vi "DSF.Transceiver.UDP.Get Transfer Group Parameters.vi"(11 "UDP Transceiver in":refnum<class "DSF.Transceiver.UDP.lvclass">) -> (2 "Transfer Group parameters":T1[](array[typedef]) {"Rx"."max size" format="%d bytes"; "Rx"."Transfers Rx"."timeout" format="%d ms"; "Rx"."Transfers Rx"."max size" format="%d bytes"}, 3 "UDP Transceiver out":refnum<class "DSF.Transceiver.UDP.lvclass">)   [LabVIEW 2017, in "DSF.Transceiver.UDP.lvlib" / "DSF.Transceiver.UDP.lvclass"]
uses:
  DSF.Transceiver.UDP.lvclass
  DSF.Transceiver.UDP.Parameters.Transfer Group.ctl
  DSF.Transceiver.UDP.Parameters.Transfer Group.Rx.ctl
  DSF.Transceiver.UDP.Parameters.Transfer.Rx.ctl
  DSF.Transceiver.UDP.Parameters.Transfer Group.Tx.ctl
  DSF.Transceiver.UDP.Parameters.Transfer.Tx.ctl
  DSF.Transceiver.UDP.lvclass/DSF.Transceiver.UDP.ctl
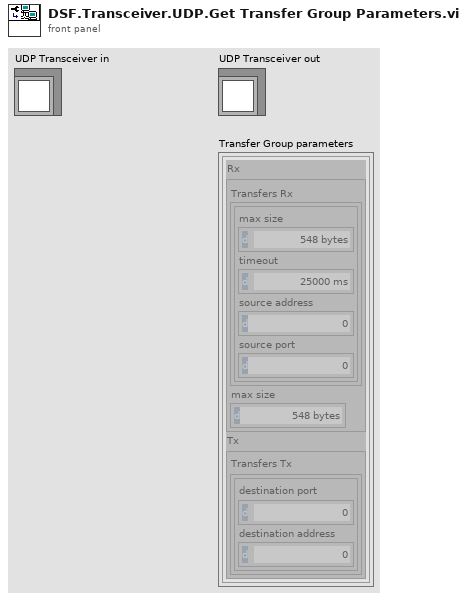
[diagram p1: front panel]
types:
  T1 = typedef "DSF.Transceiver.UDP.lvlib/DSF.Transceiver.UDP.lvclass/DSF.Transceiver.UDP.Parameters.Transfer Group.ctl" = cluster{"Rx":T2, "Tx":T4}
  T2 = typedef "DSF.Transceiver.UDP.lvlib/DSF.Transceiver.UDP.lvclass/DSF.Transceiver.UDP.Parameters.Transfer Group.Rx.ctl" = cluster{"Transfers Rx":T3[], "max size":i32}
  T3 = typedef "DSF.Transceiver.UDP.lvlib/DSF.Transceiver.UDP.lvclass/DSF.Transceiver.UDP.Parameters.Transfer.Rx.ctl" = cluster{"max size":i32, "timeout":i32, "source address":u32, "source port":u16}
  T4 = typedef "DSF.Transceiver.UDP.lvlib/DSF.Transceiver.UDP.lvclass/DSF.Transceiver.UDP.Parameters.Transfer Group.Tx.ctl" = cluster{"Transfers Tx":T5[]}
  T5 = typedef "DSF.Transceiver.UDP.lvlib/DSF.Transceiver.UDP.lvclass/DSF.Transceiver.UDP.Parameters.Transfer.Tx.ctl" = cluster{"destination port":u16, "destination address":u32}
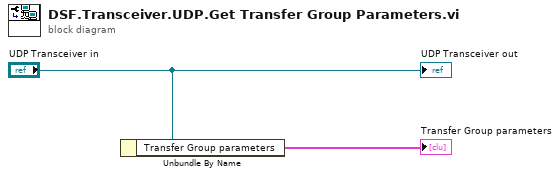
[diagram p0: block diagram]
diagram:
  n1 = Unbundle By Name("UDP Transceiver in") -> ("Transfer Group parameters"=→"Transfer Group parameters":T1[])
  "UDP Transceiver out" <- "UDP Transceiver in"
